vi "Set Target Groups (ID Array).vi"(8 "error in (no error)":errorcluster, 10 "Target Groups":T1[](array[typedef]), 11 "TCPMessaging in":refnum<class "TCPMessaging.lvclass">) -> (0 "error out":errorcluster, 3 "TCPMessaging out":refnum<class "TCPMessaging.lvclass">)   [LabVIEW 2020, in "Vecto.lvlib" / "TCPMessaging.lvclass"]
uses:
  TCPMessaging.lvclass
  Target Group.ctl
  TCPMessaging.lvclass/TCPMessaging.ctl
  Target Group Maps.ctl
  <vilib>/Utility/miscctls.llb/LVMapReplaceAction.ctl
  Vecto.lvlib
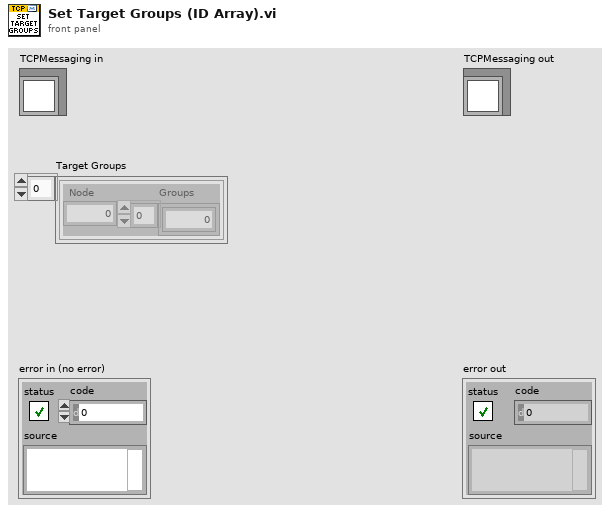
[diagram p1: front panel]
types:
  T1 = typedef "Vecto.lvlib/Target Group.ctl" = cluster{"Node":u32, "Groups":u32[]}
  T2 = typedef "Vecto.lvlib/TCPMessaging.lvclass/TCP Mode.ctl" = enum16{"Client", "Server"}
  T3 = typedef "Vecto.lvlib/TCPMessaging.lvclass/Target Group Maps.ctl" = cluster{"Target":map{u32, u32[]}, "Node":map{u32, u32[]}}
  T4 = typedef "LVMapReplaceAction.ctl" = enum32{"Modify Entry only if found", "Add or Modify Entry", "Delete Entry"}
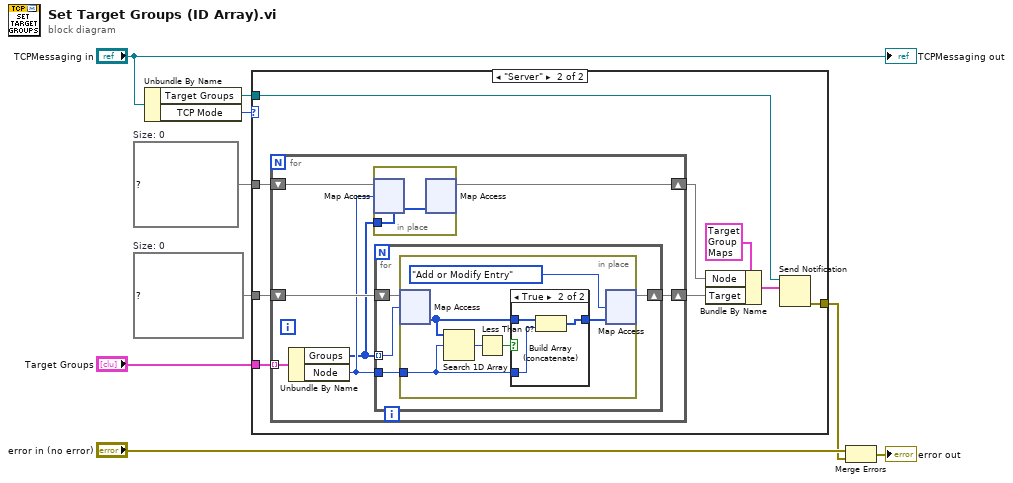
[diagram p0: block diagram]
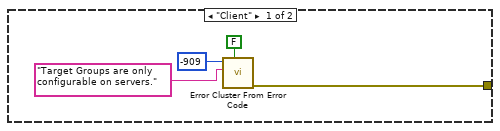
[diagram p2: hidden frame]
diagram:
  w1 = map{u32, u32[]} {}  # Size: 0
  w3 = map{u32, u32[]} {}  # Size: 0
  n1 = Unbundle By Name("TCPMessaging in") -> ("Target Groups"=w7:refnum<notifier>, "TCP Mode"=w2:T2)
  n2 = case shown="\"Server\"" w2 {
    tunnel: w7 -> [_ w22]
    tunnel: "Target Groups" -> [_ w19]
    tunnel: [w13 w21] -> w4
    tunnel: w3 -> [_ w20]
    tunnel: w1 -> [_ w18]
    frame "Client" {
      n3 = call <vilib>:"Error Cluster From Error Code.vi"("show call chain? (False)"=FALSE, "error message (\"\")"="Target Groups are only configurable on servers.", "error code (0)"=-909) -> ("error out"=w13:errorcluster)  [unwired: 6 in]
    }
    frame "Server" {
      n4 = for {
        shift-right: [w27] -> w15
        shift-left: w20 -> [w28]
        tunnel: w19 -> [w29] mode=indexing
        shift-right: [w23] -> w16
        shift-left: w18 -> [w26]
        n5 = Unbundle By Name(w29) -> ("Groups"=w24:u32[], "Node"=w25:u32)
        n6 = in-place {
          in-place-border: w24 -> [w30]
          n7 = in-place-map #1(w26, w25) -> ()  [unwired: 1 in, 2 out]
          n8 = in-place-map #1(w30) -> (w23:map{u32, u32[]})  [unwired: 1 in, 2 out]
        }
        n9 = for {
          shift-right: [w31] -> w27
          shift-left: w28 -> [w34]
          tunnel: w24 -> [w33] mode=indexing
          tunnel: w25 -> [w32]
          n10 = in-place {
            in-place-border: w32 -> [w36]
            n11 = in-place-map #2(w34, w33) -> (w38:u32[])  [unwired: 1 in, 1 out]
            n12 = Search 1D Array(1D array=w38, element=w36) -> (index of element=w39:i32)  [unwired: 1 in]
            n13 = Less Than 0?(x=w39) -> (x < 0?=w37:bool)
            n14 = case shown="True" w37 {
              tunnel: w38 -> [w41 w44]
              tunnel: w36 -> [_ w43]
              tunnel: [w41 w42] -> w35
              frame False {
              }
              frame True {
                n15 = Build Array (concatenate)(w44, w43) -> (w42:u32[])
              }
            }
            n16 = in-place-map #2(w35, LVMapReplaceAction."Add or Modify Entry" ("action")) -> (w31:map{u32, u32[]})  [unwired: 2 out]
          }
        }
      }
      n17 = Bundle By Name(cluster=T3 {"Target"={}, "Node"={}} ("Target Group Maps"), "Node"=w16, "Target"=w15) -> (w14:T3)
      n18 = Send Notification(notification=w14, notifier=w22) -> (error out=w21:errorcluster)  [unwired: 1 in, 1 out]
    }
  }
  n19 = Merge Errors("error in (no error)", w4) -> (→"error out":errorcluster)
  "TCPMessaging out" <- "TCPMessaging in"
